vi "Add Linked List.vi"(6 "Insertion Index":i32=-1, 7 "Parent ID":string, 8 "error in (no error)":errorcluster, 9 "Linked List ID":string, 10 "Name":string, 11 "Linked List Ref":refnum<data-value>) -> (0 "error out":errorcluster, 1 "Replaced?":bool, 3 "Linked List Ref out":refnum<data-value>, 5 "Linked List ID out":string)   [LabVIEW 2017, in "Linked Lists.lvlib" / "Linked List Ref.lvclass"]
uses:
  <vilib>/gpm_packages/@cs/linked-list/Source/Linked List/Linked List Ref/Linked List Ref.lvclass
  <vilib>/gpm_packages/@cs/linked-list/Source/Linked List/ILinkedList/ILinked List.lvclass
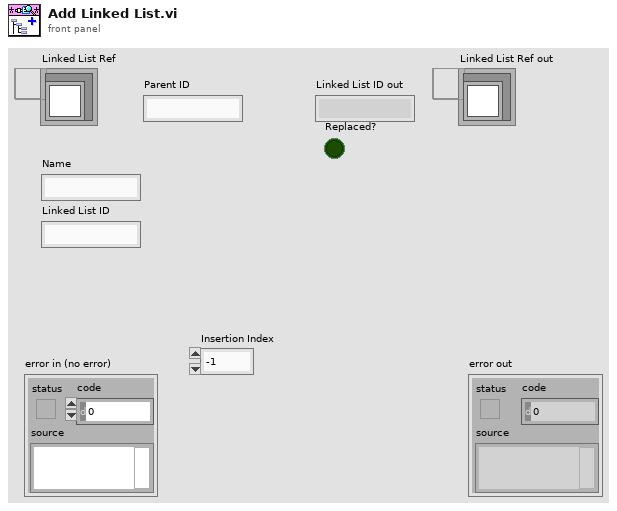
[diagram p1: front panel]
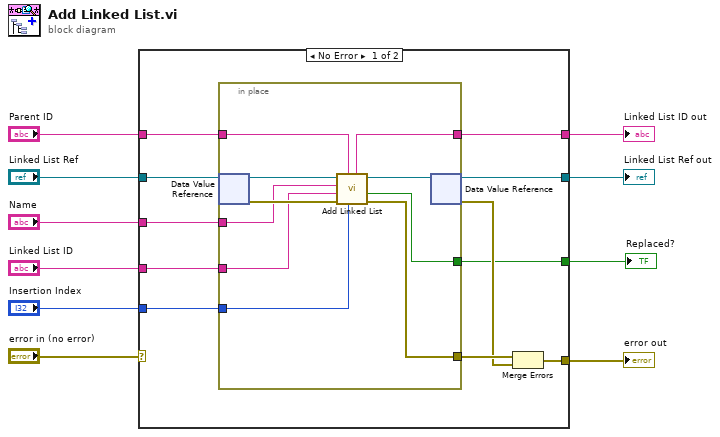
[diagram p0: block diagram]
diagram:
  n1 = case shown="No Error" "error in (no error)" {
    selector: "error in (no error)" -> [_ w33]
    tunnel: [w13 w33] -> w9
    tunnel: "Linked List Ref" -> [w20 w32]
    tunnel: [w19 w32] -> w7
    tunnel: "Parent ID" -> [w18 _]
    tunnel: [w17 _] -> w5
    tunnel: "Name" -> [w16 _]
    tunnel: "Linked List ID" -> [w15 _]
    tunnel: "Insertion Index" -> [w14 _]
    tunnel: [w11 _] -> w1
    frame No Error {
      n2 = in-place {
        in-place-border: [w31] -> w21
        in-place-border: w18 -> [w28]
        in-place-border: [w27] -> w17
        in-place-border: w16 -> [w25]
        in-place-border: w15 -> [w24]
        in-place-border: w14 -> [w23]
        in-place-border: [w22] -> w11
        n3 = in-place-dvr #1(w20) -> (w30:refnum<class "ILinked List.lvclass">, w26:errorcluster)
        n4 = call-dynamic "Add Linked List.vi"("Insertion Index"=w23, "Parent ID"=w28, "error in (no error)"=w26, "Linked List ID"=w24, "Name"=w25, "ILinked List in"=w30) -> ("error out"=w31:errorcluster, "Replaced?"=w22:bool, "ILinked List out"=w29:refnum<class "ILinked List.lvclass">, "Unique ID out"=w27:string)  [unwired: 2 in]
        n5 = in-place-dvr #1(w29) -> (w19:refnum<data-value>, w12:errorcluster)
      }
      n6 = Merge Errors(w21, w12) -> (w13:errorcluster)
    }
    frame Error {
    }
  }
  "error out" <- w9
  "Linked List Ref out" <- w7
  "Linked List ID out" <- w5
  "Replaced?" <- w1
